vi "initialization.vi"(2 "Boundary Height":i8, 3 "Boundary Width":i8) -> (0 "snake coordinates":i8[][](array[numeric]), 1 "map":bool[][](array[boolean]))   [LabVIEW 2020]
doc: "generate a display map based on the input and an array of the snake's body's cooridinate"
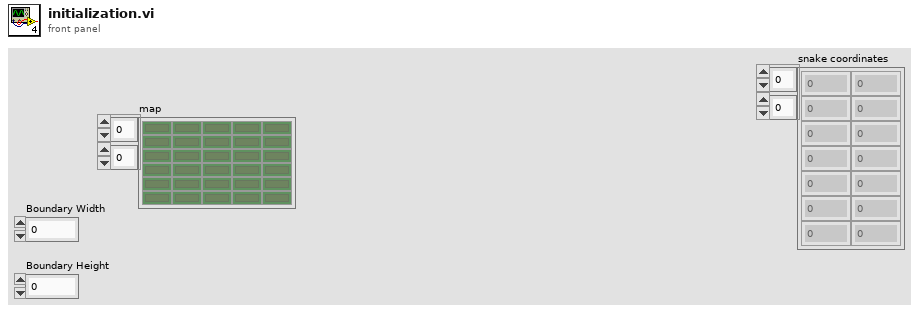
[diagram p1: front panel]
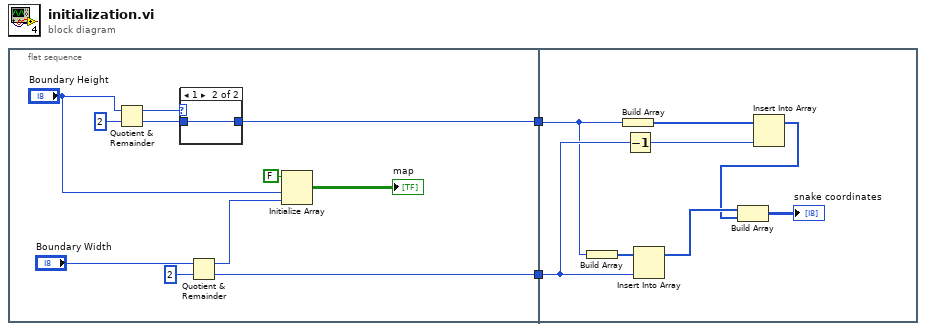
[diagram p0: block diagram]
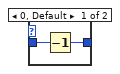
[diagram p2: hidden frame]
diagram:
  n1 = flat-sequence {
    tunnel: [w12] -> w2
    tunnel: [w8] -> w1
    tunnel: w2 -> [w19]
    tunnel: w1 -> [w18]
    frame #0 {
      n2 = Quotient & Remainder(x="Boundary Height", y=i8 2) -> (x-y*floor(x/y)=w9:i8, floor(x/y)=w7:i8)
      n3 = case shown="1" w9 {
        tunnel: [w14 w15] -> w8
        tunnel: w7 -> [w13 w15]
        frame 0, Default {
          n4 = Decrement(x=w13) -> (x-1=w14:i8)
        }
        frame 1 {
        }
      }
      n5 = Quotient & Remainder(x="Boundary Width", y=i8 2) -> (floor(x/y)=w12:i8)  [unwired: 1 out]
      n6 = Initialize Array(FALSE, "Boundary Height", "Boundary Width") -> (→"map":bool[][])
    }
    frame #1 {
      n7 = Build Array(w18) -> (w23:i8[])
      n8 = Build Array(w18) -> (w22:i8[])
      n9 = Decrement(x=w19) -> (x-1=w17:i8)
      n10 = Insert Into Array(array=w23, new element=w19) -> (w21:i8[])  [unwired: 1 in]
      n11 = Insert Into Array(array=w22, new element=w17) -> (w20:i8[])  [unwired: 1 in]
      n12 = Build Array(w21, w20) -> (→"snake coordinates":i8[][])
    }
  }
